vi "输入数据解析.vi"(0 "单个参数补充":dbl, 1 "从板号":dbl=1.0, 2 "主板二维码":string="BNET01", 3 "从板二维码":string="BNET01", 5 "主板引用":refnum<vi>, 7 "从板引用":refnum<vi>, 9 "主板选项":string="三级故障阀值", 11 "枚举":enum16{"主板", "从板"}(ring), 12 "快换":bool caption="快换写入") -> (4 "输出数组":dbl[][](array[numeric]), 6 "数组长度":dbl[](array[numeric]), 8 "循环次数":i32, 10 "命令":u32, 14 "名称":string[](array[string]), 15 "命令序号":u32[](array[numeric]))   [LabVIEW 2013] (continued)
            shift-right: [w13375] -> w13367
            shift-left: dbl[] [] -> [w13371]
            i -> [w13374]
            n5115 = case shown="2" w13374 {
              tunnel: w13373 -> [w13376 w13387 w13398 w13410 w13420 w13431 w13443 w13454]
              tunnel: [w13377 w13388 w13399 w13411 w13422 w13433 w13445 w13455] -> w13372
              frame 0, Default {
                # "最大允许单体电压"
                n5116 = disable-structure shown="启用" {
                  disable-tunnel: [w13383 w13386] -> w13379
                  disable-tunnel: [w13382 w13386] -> w13378
                  disable-tunnel: w13376 -> [w13381 _]
                  frame Disabled {
                    n5117 = Unbundle By Name(w13381) -> ("最大允许单体电压"=w13380:dbl)
                    n5118 = call "输入分辨率计算-EV05.vi"("1字节?"=FALSE, "数值"=w13380, "分辨率"=0.001) -> ("低字节"=w13382:dbl, "高字节1"=w13383:dbl)  [unwired: 2 in, 5 out]
                  }
                  frame Enabled {
                    w13386 = 255 ("高字节1")
                  }
                }
                n5119 = Build Array(w13379, w13378) -> (w13377:i32[])
              }
              frame 1 {
                # "最大允许总电压"
                n5120 = disable-structure shown="启用" {
                  disable-tunnel: [w13394 w13397] -> w13390
                  disable-tunnel: [w13393 w13397] -> w13389
                  disable-tunnel: w13387 -> [w13392 _]
                  frame Disabled {
                    n5121 = Unbundle By Name(w13392) -> ("最大允许总电压"=w13391:dbl)
                    n5122 = call "输入分辨率计算-EV05.vi"("1字节?"=FALSE, "数值"=w13391, "分辨率"=0.1) -> ("低字节"=w13393:dbl, "高字节1"=w13394:dbl)  [unwired: 2 in, 5 out]
                  }
                  frame Enabled {
                    w13397 = 255 ("高字节1")
                  }
                }
                n5123 = Build Array(w13390, w13389) -> (w13388:i32[])
              }
              frame 2 {
                # "最大允许充电电流"
                n5124 = disable-structure shown="启用" {
                  disable-tunnel: [w13406 w13409] -> w13401
                  disable-tunnel: [w13405 w13409] -> w13400
                  disable-tunnel: w13398 -> [w13403 _]
                  frame Enabled {
                    n5125 = Unbundle By Name(w13403) -> ("最大允许充电电流"=w13402:dbl)
                    n5126 = call "输入分辨率计算-EV05.vi"("1字节?"=FALSE, "数值"=w13402, "偏移量"=0.0, "分辨率"=0.1) -> ("低字节"=w13405:dbl, "高字节1"=w13406:dbl)  [unwired: 1 in, 5 out]
                  }
                  frame Disabled {
                    w13409 = 255 ("高字节1")
                  }
                }
                n5127 = Build Array(w13401, w13400) -> (w13399:dbl[])
              }
              frame 3 {
                # "最小允许充电温度"
                n5128 = disable-structure shown="启用" {
                  disable-tunnel: [w13416 255 ("高字节1")] -> w13412
                  disable-tunnel: w13410 -> [w13414 _]
                  frame Disabled {
                    n5129 = Unbundle By Name(w13414) -> ("最小允许温度"=w13413:dbl)
                    n5130 = call "输入分辨率计算-EV05.vi"("1字节?"=TRUE, "数值"=w13413, "偏移量"=-40.0, "分辨率"=1.0) -> ("高字节1"=w13416:dbl)  [unwired: 1 in, 6 out]
                  }
                  frame Enabled {
                  }
                }
                n5131 = Build Array(w13412) -> (w13411:i32[])
              }
              frame 4 {
                # "最小充电电流"
                n5132 = disable-structure shown="启用" {
                  disable-tunnel: [w13427 w13430] -> w13423
                  disable-tunnel: [w13426 w13430] -> w13421
                  disable-tunnel: w13420 -> [w13425 _]
                  frame Disabled {
                    n5133 = Unbundle By Name(w13425) -> ("最小充电电流"=w13424:dbl)
                    n5134 = call "输入分辨率计算-EV05.vi"("1字节?"=FALSE, "数值"=w13424, "分辨率"=0.1) -> ("低字节"=w13426:dbl, "高字节1"=w13427:dbl)  [unwired: 2 in, 5 out]
                  }
                  frame Enabled {
                    w13430 = 255 ("高字节1")
                  }
                }
                n5135 = Build Array(w13423, w13421) -> (w13422:i32[])
              }
              frame 5 {
                # "电流步长"
                n5136 = disable-structure shown="启用" {
                  disable-tunnel: [w13439 w13442] -> w13434
                  disable-tunnel: [w13437 w13442] -> w13432
                  disable-tunnel: w13431 -> [w13436 _]
                  frame Disabled {
                    n5137 = Unbundle By Name(w13436) -> ("电流步长"=w13435:dbl)
                    n5138 = call "输入分辨率计算-EV05.vi"("1字节?"=FALSE, "数值"=w13435, "偏移量"=0.0, "分辨率"=1.0) -> ("低字节"=w13437:dbl, "高字节1"=w13439:dbl)  [unwired: 1 in, 5 out]
                  }
                  frame Enabled {
                    w13442 = 255 ("高字节1")
                  }
                }
                n5139 = Build Array(w13434, w13432) -> (w13433:i32[])
              }
              frame 6 {
                # "最小允许单体电压"
                n5140 = disable-structure shown="启用" {
                  disable-tunnel: [w13450 w13453] -> w13446
                  disable-tunnel: [w13449 w13453] -> w13444
                  disable-tunnel: w13443 -> [w13448 _]
                  frame Disabled {
                    n5141 = Unbundle By Name(w13448) -> ("最小允许单体电压"=w13447:dbl)
                    n5142 = call "输入分辨率计算-EV05.vi"("1字节?"=FALSE, "数值"=w13447, "分辨率"=0.001) -> ("低字节"=w13449:dbl, "高字节1"=w13450:dbl)  [unwired: 2 in, 5 out]
                  }
                  frame Enabled {
                    w13453 = 255 ("高字节1")
                  }
                }
                n5143 = Build Array(w13446, w13444) -> (w13445:i32[])
              }
              frame 7 {
                # "最大允许充电温度"
                n5144 = disable-structure shown="启用" {
                  disable-tunnel: [w13460 255 ("高字节1")] -> w13456
                  disable-tunnel: w13454 -> [w13458 _]
                  frame Disabled {
                    n5145 = Unbundle By Name(w13458) -> ("最大允许充电温度"=w13457:dbl)
                    n5146 = call "输入分辨率计算-EV05.vi"("1字节?"=TRUE, "数值"=w13457, "偏移量"=-40.0, "分辨率"=1.0) -> ("高字节1"=w13460:dbl)  [unwired: 1 in, 6 out]
                  }
                  frame Enabled {
                  }
                }
                n5147 = Build Array(w13456) -> (w13455:i32[])
              }
            }
            n5148 = Insert Into Array(array=w13371, new element=w13372) -> (w13375:dbl[])  [unwired: 1 in]
          }
          n5149 = Build Array(w13367) -> (w13369:dbl[][])
        }
        frame "最小允许充电温度" {
          n5150 = Unbundle By Name(w13467) -> ("充电控制参数"=w13468:refnum<vi>)
          n5151 = property class="Clust (严格)"(reference=w13468) -> ("Value"=w13466:T6)  [unwired: 1 in, 2 out]
          n5152 = for {
            N: 8 -> [_]
            tunnel: w13466 -> [w13478]
            shift-right: [w13480] -> w13472
            shift-left: dbl[] [] -> [w13476]
            i -> [w13479]
            n5153 = case shown="3" w13479 {
              tunnel: w13478 -> [w13481 w13492 w13503 w13515 w13525 w13536 w13548 w13559]
              tunnel: [w13482 w13493 w13504 w13516 w13527 w13538 w13550 w13560] -> w13477
              frame 0, Default {
                # "最大允许单体电压"
                n5154 = disable-structure shown="启用" {
                  disable-tunnel: [w13488 w13491] -> w13484
                  disable-tunnel: [w13487 w13491] -> w13483
                  disable-tunnel: w13481 -> [w13486 _]
                  frame Disabled {
                    n5155 = Unbundle By Name(w13486) -> ("最大允许单体电压"=w13485:dbl)
                    n5156 = call "输入分辨率计算-EV05.vi"("1字节?"=FALSE, "数值"=w13485, "分辨率"=0.001) -> ("低字节"=w13487:dbl, "高字节1"=w13488:dbl)  [unwired: 2 in, 5 out]
                  }
                  frame Enabled {
                    w13491 = 255 ("高字节1")
                  }
                }
                n5157 = Build Array(w13484, w13483) -> (w13482:i32[])
              }
              frame 1 {
                # "最大允许总电压"
                n5158 = disable-structure shown="启用" {
                  disable-tunnel: [w13499 w13502] -> w13495
                  disable-tunnel: [w13498 w13502] -> w13494
                  disable-tunnel: w13492 -> [w13497 _]
                  frame Disabled {
                    n5159 = Unbundle By Name(w13497) -> ("最大允许总电压"=w13496:dbl)
                    n5160 = call "输入分辨率计算-EV05.vi"("1字节?"=FALSE, "数值"=w13496, "分辨率"=0.1) -> ("低字节"=w13498:dbl, "高字节1"=w13499:dbl)  [unwired: 2 in, 5 out]
                  }
                  frame Enabled {
                    w13502 = 255 ("高字节1")
                  }
                }
                n5161 = Build Array(w13495, w13494) -> (w13493:i32[])
              }
              frame 2 {
                # "最大允许充电电流"
                n5162 = disable-structure shown="启用" {
                  disable-tunnel: [w13511 w13514] -> w13506
                  disable-tunnel: [w13510 w13514] -> w13505
                  disable-tunnel: w13503 -> [w13508 _]
                  frame Disabled {
                    n5163 = Unbundle By Name(w13508) -> ("最大允许充电电流"=w13507:dbl)
                    n5164 = call "输入分辨率计算-EV05.vi"("1字节?"=FALSE, "数值"=w13507, "偏移量"=-3000.0, "分辨率"=0.1) -> ("低字节"=w13510:dbl, "高字节1"=w13511:dbl)  [unwired: 1 in, 5 out]
                  }
                  frame Enabled {
                    w13514 = 255 ("高字节1")
                  }
                }
                n5165 = Build Array(w13506, w13505) -> (w13504:i32[])
              }
              frame 3 {
                # "最小允许充电温度"
                n5166 = disable-structure shown="启用" {
                  disable-tunnel: [w13521 255 ("高字节1")] -> w13517
                  disable-tunnel: w13515 -> [w13519 _]
                  frame Enabled {
                    n5167 = Unbundle By Name(w13519) -> ("最小允许充电温度"=w13518:dbl)
                    n5168 = call "输入分辨率计算-EV05.vi"("1字节?"=TRUE, "数值"=w13518, "偏移量"=-40.0, "分辨率"=1.0) -> ("高字节1"=w13521:dbl)  [unwired: 1 in, 6 out]
                  }
                  frame Disabled {
                  }
                }
                n5169 = Build Array(w13517) -> (w13516:dbl[])
              }
              frame 4 {
                # "最小充电电流"
                n5170 = disable-structure shown="启用" {
                  disable-tunnel: [w13532 w13535] -> w13528
                  disable-tunnel: [w13531 w13535] -> w13526
                  disable-tunnel: w13525 -> [w13530 _]
                  frame Disabled {
                    n5171 = Unbundle By Name(w13530) -> ("最小充电电流"=w13529:dbl)
                    n5172 = call "输入分辨率计算-EV05.vi"("1字节?"=FALSE, "数值"=w13529, "分辨率"=0.1) -> ("低字节"=w13531:dbl, "高字节1"=w13532:dbl)  [unwired: 2 in, 5 out]
                  }
                  frame Enabled {
                    w13535 = 255 ("高字节1")
                  }
                }
                n5173 = Build Array(w13528, w13526) -> (w13527:i32[])
              }
              frame 5 {
                # "电流步长"
                n5174 = disable-structure shown="启用" {
                  disable-tunnel: [w13544 w13547] -> w13539
                  disable-tunnel: [w13542 w13547] -> w13537
                  disable-tunnel: w13536 -> [w13541 _]
                  frame Disabled {
                    n5175 = Unbundle By Name(w13541) -> ("电流步长"=w13540:dbl)
                    n5176 = call "输入分辨率计算-EV05.vi"("1字节?"=FALSE, "数值"=w13540, "偏移量"=0.0, "分辨率"=1.0) -> ("低字节"=w13542:dbl, "高字节1"=w13544:dbl)  [unwired: 1 in, 5 out]
                  }
                  frame Enabled {
                    w13547 = 255 ("高字节1")
                  }
                }
                n5177 = Build Array(w13539, w13537) -> (w13538:i32[])
              }
              frame 6 {
                # "最小允许单体电压"
                n5178 = disable-structure shown="启用" {
                  disable-tunnel: [w13555 w13558] -> w13551
                  disable-tunnel: [w13554 w13558] -> w13549
                  disable-tunnel: w13548 -> [w13553 _]
                  frame Disabled {
                    n5179 = Unbundle By Name(w13553) -> ("最小允许单体电压"=w13552:dbl)
                    n5180 = call "输入分辨率计算-EV05.vi"("1字节?"=FALSE, "数值"=w13552, "分辨率"=0.001) -> ("低字节"=w13554:dbl, "高字节1"=w13555:dbl)  [unwired: 2 in, 5 out]
                  }
                  frame Enabled {
                    w13558 = 255 ("高字节1")
                  }
                }
                n5181 = Build Array(w13551, w13549) -> (w13550:i32[])
              }
              frame 7 {
                # "最大允许充电温度"
                n5182 = disable-structure shown="启用" {
                  disable-tunnel: [w13565 255 ("高字节1")] -> w13561
                  disable-tunnel: w13559 -> [w13563 _]
                  frame Disabled {
                    n5183 = Unbundle By Name(w13563) -> ("最大允许充电温度"=w13562:dbl)
                    n5184 = call "输入分辨率计算-EV05.vi"("1字节?"=TRUE, "数值"=w13562, "偏移量"=-40.0, "分辨率"=1.0) -> ("高字节1"=w13565:dbl)  [unwired: 1 in, 6 out]
                  }
                  frame Enabled {
                  }
                }
                n5185 = Build Array(w13561) -> (w13560:i32[])
              }
            }
            n5186 = Insert Into Array(array=w13476, new element=w13477) -> (w13480:dbl[])  [unwired: 1 in]
          }
          n5187 = Build Array(w13472) -> (w13474:dbl[][])
        }
        frame "最小允许充电电流" {
          n5188 = Unbundle By Name(w13572) -> ("充电控制参数"=w13573:refnum<vi>)
          n5189 = property class="Clust (严格)"(reference=w13573) -> ("Value"=w13571:T6)  [unwired: 1 in, 2 out]
          n5190 = for {
            N: 8 -> [_]
            tunnel: w13571 -> [w13583]
            shift-right: [w13585] -> w13577
            shift-left: dbl[] [] -> [w13581]
            i -> [w13584]
            n5191 = case shown="4" w13584 {
              tunnel: w13583 -> [w13586 w13597 w13608 w13620 w13630 w13641 w13653 w13664]
              tunnel: [w13587 w13598 w13609 w13621 w13632 w13643 w13655 w13665] -> w13582
              frame 0, Default {
                # "最大允许单体电压"
                n5192 = disable-structure shown="启用" {
                  disable-tunnel: [w13593 w13596] -> w13589
                  disable-tunnel: [w13592 w13596] -> w13588
                  disable-tunnel: w13586 -> [w13591 _]
                  frame Disabled {
                    n5193 = Unbundle By Name(w13591) -> ("最大允许单体电压"=w13590:dbl)
                    n5194 = call "输入分辨率计算-EV05.vi"("1字节?"=FALSE, "数值"=w13590, "分辨率"=0.001) -> ("低字节"=w13592:dbl, "高字节1"=w13593:dbl)  [unwired: 2 in, 5 out]
                  }
                  frame Enabled {
                    w13596 = 255 ("高字节1")
                  }
                }
                n5195 = Build Array(w13589, w13588) -> (w13587:i32[])
              }
              frame 1 {
                # "最大允许总电压"
                n5196 = disable-structure shown="启用" {
                  disable-tunnel: [w13604 w13607] -> w13600
                  disable-tunnel: [w13603 w13607] -> w13599
                  disable-tunnel: w13597 -> [w13602 _]
                  frame Disabled {
                    n5197 = Unbundle By Name(w13602) -> ("最大允许总电压"=w13601:dbl)
                    n5198 = call "输入分辨率计算-EV05.vi"("1字节?"=FALSE, "数值"=w13601, "分辨率"=0.1) -> ("低字节"=w13603:dbl, "高字节1"=w13604:dbl)  [unwired: 2 in, 5 out]
                  }
                  frame Enabled {
                    w13607 = 255 ("高字节1")
                  }
                }
                n5199 = Build Array(w13600, w13599) -> (w13598:i32[])
              }
              frame 2 {
                # "最大允许充电电流"
                n5200 = disable-structure shown="启用" {
                  disable-tunnel: [w13616 w13619] -> w13611
                  disable-tunnel: [w13615 w13619] -> w13610
                  disable-tunnel: w13608 -> [w13613 _]
                  frame Disabled {
                    n5201 = Unbundle By Name(w13613) -> ("最大允许充电电流"=w13612:dbl)
                    n5202 = call "输入分辨率计算-EV05.vi"("1字节?"=FALSE, "数值"=w13612, "偏移量"=-3000.0, "分辨率"=0.1) -> ("低字节"=w13615:dbl, "高字节1"=w13616:dbl)  [unwired: 1 in, 5 out]
                  }
                  frame Enabled {
                    w13619 = 255 ("高字节1")
                  }
                }
                n5203 = Build Array(w13611, w13610) -> (w13609:i32[])
              }
              frame 3 {
                # "最小允许充电温度"
                n5204 = disable-structure shown="启用" {
                  disable-tunnel: [w13626 255 ("高字节1")] -> w13622
                  disable-tunnel: w13620 -> [w13624 _]
                  frame Disabled {
                    n5205 = Unbundle By Name(w13624) -> ("最小允许温度"=w13623:dbl)
                    n5206 = call "输入分辨率计算-EV05.vi"("1字节?"=TRUE, "数值"=w13623, "偏移量"=-40.0, "分辨率"=1.0) -> ("高字节1"=w13626:dbl)  [unwired: 1 in, 6 out]
                  }
                  frame Enabled {
                  }
                }
                n5207 = Build Array(w13622) -> (w13621:i32[])
              }
              frame 4 {
                # "最小充电电流"
                n5208 = disable-structure shown="启用" {
                  disable-tunnel: [w13637 w13640] -> w13633
                  disable-tunnel: [w13636 w13640] -> w13631
                  disable-tunnel: w13630 -> [w13635 _]
                  frame Enabled {
                    n5209 = Unbundle By Name(w13635) -> ("最小允许充电电流"=w13634:dbl)
                    n5210 = call "输入分辨率计算-EV05.vi"("1字节?"=FALSE, "数值"=w13634, "分辨率"=0.1) -> ("低字节"=w13636:dbl, "高字节1"=w13637:dbl)  [unwired: 2 in, 5 out]
                  }
                  frame Disabled {
                    w13640 = 255 ("高字节1")
                  }
                }
                n5211 = Build Array(w13633, w13631) -> (w13632:dbl[])
              }
              frame 5 {
                # "电流步长"
                n5212 = disable-structure shown="启用" {
                  disable-tunnel: [w13649 w13652] -> w13644
                  disable-tunnel: [w13647 w13652] -> w13642
                  disable-tunnel: w13641 -> [w13646 _]
                  frame Disabled {
                    n5213 = Unbundle By Name(w13646) -> ("电流步长"=w13645:dbl)
                    n5214 = call "输入分辨率计算-EV05.vi"("1字节?"=FALSE, "数值"=w13645, "偏移量"=0.0, "分辨率"=1.0) -> ("低字节"=w13647:dbl, "高字节1"=w13649:dbl)  [unwired: 1 in, 5 out]
                  }
                  frame Enabled {
                    w13652 = 255 ("高字节1")
                  }
                }
                n5215 = Build Array(w13644, w13642) -> (w13643:i32[])
              }
              frame 6 {
                # "最小允许单体电压"
                n5216 = disable-structure shown="启用" {
                  disable-tunnel: [w13660 w13663] -> w13656
                  disable-tunnel: [w13659 w13663] -> w13654
                  disable-tunnel: w13653 -> [w13658 _]
                  frame Disabled {
                    n5217 = Unbundle By Name(w13658) -> ("最小允许单体电压"=w13657:dbl)
                    n5218 = call "输入分辨率计算-EV05.vi"("1字节?"=FALSE, "数值"=w13657, "分辨率"=0.001) -> ("低字节"=w13659:dbl, "高字节1"=w13660:dbl)  [unwired: 2 in, 5 out]
                  }
                  frame Enabled {
                    w13663 = 255 ("高字节1")
                  }
                }
                n5219 = Build Array(w13656, w13654) -> (w13655:i32[])
              }
              frame 7 {
                # "最大允许充电温度"
                n5220 = disable-structure shown="启用" {
                  disable-tunnel: [w13670 255 ("高字节1")] -> w13666
                  disable-tunnel: w13664 -> [w13668 _]
                  frame Disabled {
                    n5221 = Unbundle By Name(w13668) -> ("最大允许充电温度"=w13667:dbl)
                    n5222 = call "输入分辨率计算-EV05.vi"("1字节?"=TRUE, "数值"=w13667, "偏移量"=-40.0, "分辨率"=1.0) -> ("高字节1"=w13670:dbl)  [unwired: 1 in, 6 out]
                  }
                  frame Enabled {
                  }
                }
                n5223 = Build Array(w13666) -> (w13665:i32[])
              }
            }
            n5224 = Insert Into Array(array=w13581, new element=w13582) -> (w13585:dbl[])  [unwired: 1 in]
          }
          n5225 = Build Array(w13577) -> (w13579:dbl[][])
        }
        frame "电流步长" {
          n5226 = Unbundle By Name(w13677) -> ("充电控制参数"=w13678:refnum<vi>)
          n5227 = property class="Clust (严格)"(reference=w13678) -> ("Value"=w13676:T6)  [unwired: 1 in, 2 out]
          n5228 = for {
            N: 8 -> [_]
            tunnel: w13676 -> [w13688]
            shift-right: [w13690] -> w13682
            shift-left: dbl[] [] -> [w13686]
            i -> [w13689]
            n5229 = case shown="5" w13689 {
              tunnel: w13688 -> [w13691 w13702 w13713 w13725 w13735 w13746 w13758 w13769]
              tunnel: [w13692 w13703 w13714 w13726 w13737 w13748 w13760 w13770] -> w13687
              frame 0, Default {
                # "最大允许单体电压"
                n5230 = disable-structure shown="启用" {
                  disable-tunnel: [w13698 w13701] -> w13694
                  disable-tunnel: [w13697 w13701] -> w13693
                  disable-tunnel: w13691 -> [w13696 _]
                  frame Disabled {
                    n5231 = Unbundle By Name(w13696) -> ("最大允许单体电压"=w13695:dbl)
                    n5232 = call "输入分辨率计算-EV05.vi"("1字节?"=FALSE, "数值"=w13695, "分辨率"=0.001) -> ("低字节"=w13697:dbl, "高字节1"=w13698:dbl)  [unwired: 2 in, 5 out]
                  }
                  frame Enabled {
                    w13701 = 255 ("高字节1")
                  }
                }
                n5233 = Build Array(w13694, w13693) -> (w13692:i32[])
              }
              frame 1 {
                # "最大允许总电压"
                n5234 = disable-structure shown="启用" {
                  disable-tunnel: [w13709 w13712] -> w13705
                  disable-tunnel: [w13708 w13712] -> w13704
                  disable-tunnel: w13702 -> [w13707 _]
                  frame Disabled {
                    n5235 = Unbundle By Name(w13707) -> ("最大允许总电压"=w13706:dbl)
                    n5236 = call "输入分辨率计算-EV05.vi"("1字节?"=FALSE, "数值"=w13706, "分辨率"=0.1) -> ("低字节"=w13708:dbl, "高字节1"=w13709:dbl)  [unwired: 2 in, 5 out]
                  }
                  frame Enabled {
                    w13712 = 255 ("高字节1")
                  }
                }
                n5237 = Build Array(w13705, w13704) -> (w13703:i32[])
              }
              frame 2 {
                # "最大允许充电电流"
                n5238 = disable-structure shown="启用" {
                  disable-tunnel: [w13721 w13724] -> w13716
                  disable-tunnel: [w13720 w13724] -> w13715
                  disable-tunnel: w13713 -> [w13718 _]
                  frame Disabled {
                    n5239 = Unbundle By Name(w13718) -> ("最大允许充电电流"=w13717:dbl)
                    n5240 = call "输入分辨率计算-EV05.vi"("1字节?"=FALSE, "数值"=w13717, "偏移量"=-3000.0, "分辨率"=0.1) -> ("低字节"=w13720:dbl, "高字节1"=w13721:dbl)  [unwired: 1 in, 5 out]
                  }
                  frame Enabled {
                    w13724 = 255 ("高字节1")
                  }
                }
                n5241 = Build Array(w13716, w13715) -> (w13714:i32[])
              }
              frame 3 {
                # "最小允许充电温度"
                n5242 = disable-structure shown="启用" {
                  disable-tunnel: [w13731 255 ("高字节1")] -> w13727
                  disable-tunnel: w13725 -> [w13729 _]
                  frame Disabled {
                    n5243 = Unbundle By Name(w13729) -> ("最小允许温度"=w13728:dbl)
                    n5244 = call "输入分辨率计算-EV05.vi"("1字节?"=TRUE, "数值"=w13728, "偏移量"=-40.0, "分辨率"=1.0) -> ("高字节1"=w13731:dbl)  [unwired: 1 in, 6 out]
                  }
                  frame Enabled {
                  }
                }
                n5245 = Build Array(w13727) -> (w13726:i32[])
              }
              frame 4 {
                # "最小充电电流"
                n5246 = disable-structure shown="启用" {
                  disable-tunnel: [w13742 w13745] -> w13738
                  disable-tunnel: [w13741 w13745] -> w13736
                  disable-tunnel: w13735 -> [w13740 _]
                  frame Disabled {
                    n5247 = Unbundle By Name(w13740) -> ("最小充电电流"=w13739:dbl)
                    n5248 = call "输入分辨率计算-EV05.vi"("1字节?"=FALSE, "数值"=w13739, "分辨率"=0.1) -> ("低字节"=w13741:dbl, "高字节1"=w13742:dbl)  [unwired: 2 in, 5 out]
                  }
                  frame Enabled {
                    w13745 = 255 ("高字节1")
                  }
                }
                n5249 = Build Array(w13738, w13736) -> (w13737:i32[])
              }
              frame 5 {
                # "电流步长"
                n5250 = disable-structure shown="启用" {
                  disable-tunnel: [w13754 w13757] -> w13749
                  disable-tunnel: [w13752 w13757] -> w13747
                  disable-tunnel: w13746 -> [w13751 _]
                  frame Enabled {
                    n5251 = Unbundle By Name(w13751) -> ("电流步长"=w13750:dbl)
                    n5252 = call "输入分辨率计算-EV05.vi"("1字节?"=FALSE, "数值"=w13750, "偏移量"=0.0, "分辨率"=0.1) -> ("低字节"=w13752:dbl, "高字节1"=w13754:dbl)  [unwired: 1 in, 5 out]
                  }
                  frame Disabled {
                    w13757 = 255 ("高字节1")
                  }
                }
                n5253 = Build Array(w13749, w13747) -> (w13748:dbl[])
              }
              frame 6 {
                # "最小允许单体电压"
                n5254 = disable-structure shown="启用" {
                  disable-tunnel: [w13765 w13768] -> w13761
                  disable-tunnel: [w13764 w13768] -> w13759
                  disable-tunnel: w13758 -> [w13763 _]
                  frame Disabled {
                    n5255 = Unbundle By Name(w13763) -> ("最小允许单体电压"=w13762:dbl)
                    n5256 = call "输入分辨率计算-EV05.vi"("1字节?"=FALSE, "数值"=w13762, "分辨率"=0.001) -> ("低字节"=w13764:dbl, "高字节1"=w13765:dbl)  [unwired: 2 in, 5 out]
                  }
                  frame Enabled {
                    w13768 = 255 ("高字节1")
                  }
                }
                n5257 = Build Array(w13761, w13759) -> (w13760:i32[])
              }
              frame 7 {
                # "最大允许充电温度"
                n5258 = disable-structure shown="启用" {
                  disable-tunnel: [w13775 255 ("高字节1")] -> w13771
                  disable-tunnel: w13769 -> [w13773 _]
                  frame Disabled {
                    n5259 = Unbundle By Name(w13773) -> ("最大允许充电温度"=w13772:dbl)
                    n5260 = call "输入分辨率计算-EV05.vi"("1字节?"=TRUE, "数值"=w13772, "偏移量"=-40.0, "分辨率"=1.0) -> ("高字节1"=w13775:dbl)  [unwired: 1 in, 6 out]
                  }
                  frame Enabled {
                  }
                }
                n5261 = Build Array(w13771) -> (w13770:i32[])
              }
            }
            n5262 = Insert Into Array(array=w13686, new element=w13687) -> (w13690:dbl[])  [unwired: 1 in]
          }
          n5263 = Build Array(w13682) -> (w13684:dbl[][])
        }
        frame "最小允许单体电压" {
          n5264 = Unbundle By Name(w13782) -> ("充电控制参数"=w13783:refnum<vi>)
          n5265 = property class="Clust (严格)"(reference=w13783) -> ("Value"=w13781:T6)  [unwired: 1 in, 2 out]
          n5266 = for {
            N: 8 -> [_]
            tunnel: w13781 -> [w13793]
            shift-right: [w13795] -> w13787
            shift-left: dbl[] [] -> [w13791]
            i -> [w13794]
            n5267 = case shown="6" w13794 {
              tunnel: w13793 -> [w13796 w13807 w13818 w13830 w13840 w13851 w13863 w13874]
              tunnel: [w13797 w13808 w13819 w13831 w13842 w13853 w13865 w13875] -> w13792
              frame 0, Default {
                # "最大允许单体电压"
                n5268 = disable-structure shown="启用" {
                  disable-tunnel: [w13803 w13806] -> w13799
                  disable-tunnel: [w13802 w13806] -> w13798
                  disable-tunnel: w13796 -> [w13801 _]
                  frame Disabled {
                    n5269 = Unbundle By Name(w13801) -> ("最大允许单体电压"=w13800:dbl)
                    n5270 = call "输入分辨率计算-EV05.vi"("1字节?"=FALSE, "数值"=w13800, "分辨率"=0.001) -> ("低字节"=w13802:dbl, "高字节1"=w13803:dbl)  [unwired: 2 in, 5 out]
                  }
                  frame Enabled {
                    w13806 = 255 ("高字节1")
                  }
                }
                n5271 = Build Array(w13799, w13798) -> (w13797:i32[])
              }
              frame 1 {
                # "最大允许总电压"
                n5272 = disable-structure shown="启用" {
                  disable-tunnel: [w13814 w13817] -> w13810
                  disable-tunnel: [w13813 w13817] -> w13809
                  disable-tunnel: w13807 -> [w13812 _]
                  frame Disabled {
                    n5273 = Unbundle By Name(w13812) -> ("最大允许总电压"=w13811:dbl)
                    n5274 = call "输入分辨率计算-EV05.vi"("1字节?"=FALSE, "数值"=w13811, "分辨率"=0.1) -> ("低字节"=w13813:dbl, "高字节1"=w13814:dbl)  [unwired: 2 in, 5 out]
                  }
                  frame Enabled {
                    w13817 = 255 ("高字节1")
                  }
                }
                n5275 = Build Array(w13810, w13809) -> (w13808:i32[])
              }
              frame 2 {
                # "最大允许充电电流"
                n5276 = disable-structure shown="启用" {
                  disable-tunnel: [w13826 w13829] -> w13821
                  disable-tunnel: [w13825 w13829] -> w13820
                  disable-tunnel: w13818 -> [w13823 _]
                  frame Disabled {
                    n5277 = Unbundle By Name(w13823) -> ("最大允许充电电流"=w13822:dbl)
                    n5278 = call "输入分辨率计算-EV05.vi"("1字节?"=FALSE, "数值"=w13822, "偏移量"=-3000.0, "分辨率"=0.1) -> ("低字节"=w13825:dbl, "高字节1"=w13826:dbl)  [unwired: 1 in, 5 out]
                  }
                  frame Enabled {
                    w13829 = 255 ("高字节1")
                  }
                }
                n5279 = Build Array(w13821, w13820) -> (w13819:i32[])
              }
              frame 3 {
                # "最小允许充电温度"
                n5280 = disable-structure shown="启用" {
                  disable-tunnel: [w13836 255 ("高字节1")] -> w13832
                  disable-tunnel: w13830 -> [w13834 _]
                  frame Disabled {
                    n5281 = Unbundle By Name(w13834) -> ("最小允许温度"=w13833:dbl)
                    n5282 = call "输入分辨率计算-EV05.vi"("1字节?"=TRUE, "数值"=w13833, "偏移量"=-40.0, "分辨率"=1.0) -> ("高字节1"=w13836:dbl)  [unwired: 1 in, 6 out]
                  }
                  frame Enabled {
                  }
                }
                n5283 = Build Array(w13832) -> (w13831:i32[])
              }
              frame 4 {
                # "最小充电电流"
                n5284 = disable-structure shown="启用" {
                  disable-tunnel: [w13847 w13850] -> w13843
                  disable-tunnel: [w13846 w13850] -> w13841
                  disable-tunnel: w13840 -> [w13845 _]
                  frame Disabled {
                    n5285 = Unbundle By Name(w13845) -> ("最小充电电流"=w13844:dbl)
                    n5286 = call "输入分辨率计算-EV05.vi"("1字节?"=FALSE, "数值"=w13844, "分辨率"=0.1) -> ("低字节"=w13846:dbl, "高字节1"=w13847:dbl)  [unwired: 2 in, 5 out]
                  }
                  frame Enabled {
                    w13850 = 255 ("高字节1")
                  }
                }
                n5287 = Build Array(w13843, w13841) -> (w13842:i32[])
              }
              frame 5 {
                # "电流步长"
                n5288 = disable-structure shown="启用" {
                  disable-tunnel: [w13859 w13862] -> w13854
                  disable-tunnel: [w13857 w13862] -> w13852
                  disable-tunnel: w13851 -> [w13856 _]
                  frame Disabled {
                    n5289 = Unbundle By Name(w13856) -> ("电流步长"=w13855:dbl)
                    n5290 = call "输入分辨率计算-EV05.vi"("1字节?"=FALSE, "数值"=w13855, "偏移量"=0.0, "分辨率"=1.0) -> ("低字节"=w13857:dbl, "高字节1"=w13859:dbl)  [unwired: 1 in, 5 out]
                  }
                  frame Enabled {
                    w13862 = 255 ("高字节1")
                  }
                }
                n5291 = Build Array(w13854, w13852) -> (w13853:i32[])
              }
              frame 6 {
                # "最小允许单体电压"
                n5292 = disable-structure shown="启用" {
                  disable-tunnel: [w13870 w13873] -> w13866
                  disable-tunnel: [w13869 w13873] -> w13864
                  disable-tunnel: w13863 -> [w13868 _]
                  frame Enabled {
                    n5293 = Unbundle By Name(w13868) -> ("最小允许单体电压"=w13867:dbl)
                    n5294 = call "输入分辨率计算-EV05.vi"("1字节?"=FALSE, "数值"=w13867, "分辨率"=0.001) -> ("低字节"=w13869:dbl, "高字节1"=w13870:dbl)  [unwired: 2 in, 5 out]
                  }
                  frame Disabled {
                    w13873 = 255 ("高字节1")
                  }
                }
                n5295 = Build Array(w13866, w13864) -> (w13865:dbl[])
              }
              frame 7 {
                # "最大允许充电温度"
                n5296 = disable-structure shown="启用" {
                  disable-tunnel: [w13880 255 ("高字节1")] -> w13876
                  disable-tunnel: w13874 -> [w13878 _]
                  frame Disabled {
                    n5297 = Unbundle By Name(w13878) -> ("最大允许充电温度"=w13877:dbl)
                    n5298 = call "输入分辨率计算-EV05.vi"("1字节?"=TRUE, "数值"=w13877, "偏移量"=-40.0, "分辨率"=1.0) -> ("高字节1"=w13880:dbl)  [unwired: 1 in, 6 out]
                  }
                  frame Enabled {
                  }
                }
                n5299 = Build Array(w13876) -> (w13875:i32[])
              }
            }
            n5300 = Insert Into Array(array=w13791, new element=w13792) -> (w13795:dbl[])  [unwired: 1 in]
          }
          n5301 = Build Array(w13787) -> (w13789:dbl[][])
        }
        frame "最大允许充电温度" {
          n5302 = Unbundle By Name(w13887) -> ("充电控制参数"=w13888:refnum<vi>)
          n5303 = property class="Clust (严格)"(reference=w13888) -> ("Value"=w13886:T6)  [unwired: 1 in, 2 out]
          n5304 = for {
            N: 8 -> [_]
            tunnel: w13886 -> [w13898]
            shift-right: [w13900] -> w13892
            shift-left: dbl[] [] -> [w13896]
            i -> [w13899]
            n5305 = case shown="7" w13899 {
              tunnel: w13898 -> [w13901 w13912 w13923 w13935 w13945 w13956 w13968 w13979]
              tunnel: [w13902 w13913 w13924 w13936 w13947 w13958 w13970 w13980] -> w13897
              frame 0, Default {
                # "最大允许单体电压"
                n5306 = disable-structure shown="启用" {
                  disable-tunnel: [w13908 w13911] -> w13904
                  disable-tunnel: [w13907 w13911] -> w13903
                  disable-tunnel: w13901 -> [w13906 _]
                  frame Disabled {
                    n5307 = Unbundle By Name(w13906) -> ("最大允许单体电压"=w13905:dbl)
                    n5308 = call "输入分辨率计算-EV05.vi"("1字节?"=FALSE, "数值"=w13905, "分辨率"=0.001) -> ("低字节"=w13907:dbl, "高字节1"=w13908:dbl)  [unwired: 2 in, 5 out]
                  }
                  frame Enabled {
                    w13911 = 255 ("高字节1")
                  }
                }
                n5309 = Build Array(w13904, w13903) -> (w13902:i32[])
              }
              frame 1 {
                # "最大允许总电压"
                n5310 = disable-structure shown="启用" {
                  disable-tunnel: [w13919 w13922] -> w13915
                  disable-tunnel: [w13918 w13922] -> w13914
                  disable-tunnel: w13912 -> [w13917 _]
                  frame Disabled {
                    n5311 = Unbundle By Name(w13917) -> ("最大允许总电压"=w13916:dbl)
                    n5312 = call "输入分辨率计算-EV05.vi"("1字节?"=FALSE, "数值"=w13916, "分辨率"=0.1) -> ("低字节"=w13918:dbl, "高字节1"=w13919:dbl)  [unwired: 2 in, 5 out]
                  }
                  frame Enabled {
                    w13922 = 255 ("高字节1")
                  }
                }
                n5313 = Build Array(w13915, w13914) -> (w13913:i32[])
              }
              frame 2 {
                # "最大允许充电电流"
                n5314 = disable-structure shown="启用" {
                  disable-tunnel: [w13931 w13934] -> w13926
                  disable-tunnel: [w13930 w13934] -> w13925
                  disable-tunnel: w13923 -> [w13928 _]
                  frame Disabled {
                    n5315 = Unbundle By Name(w13928) -> ("最大允许充电电流"=w13927:dbl)
                    n5316 = call "输入分辨率计算-EV05.vi"("1字节?"=FALSE, "数值"=w13927, "偏移量"=-3000.0, "分辨率"=0.1) -> ("低字节"=w13930:dbl, "高字节1"=w13931:dbl)  [unwired: 1 in, 5 out]
                  }
                  frame Enabled {
                    w13934 = 255 ("高字节1")
                  }
                }
                n5317 = Build Array(w13926, w13925) -> (w13924:i32[])
              }
              frame 3 {
                # "最小允许充电温度"
                n5318 = disable-structure shown="启用" {
                  disable-tunnel: [w13941 255 ("高字节1")] -> w13937
                  disable-tunnel: w13935 -> [w13939 _]
                  frame Disabled {
                    n5319 = Unbundle By Name(w13939) -> ("最小允许温度"=w13938:dbl)
                    n5320 = call "输入分辨率计算-EV05.vi"("1字节?"=TRUE, "数值"=w13938, "偏移量"=-40.0, "分辨率"=1.0) -> ("高字节1"=w13941:dbl)  [unwired: 1 in, 6 out]
                  }
                  frame Enabled {
                  }
                }
                n5321 = Build Array(w13937) -> (w13936:i32[])
              }
              frame 4 {
                # "最小充电电流"
                n5322 = disable-structure shown="启用" {
                  disable-tunnel: [w13952 w13955] -> w13948
                  disable-tunnel: [w13951 w13955] -> w13946
                  disable-tunnel: w13945 -> [w13950 _]
                  frame Disabled {
                    n5323 = Unbundle By Name(w13950) -> ("最小充电电流"=w13949:dbl)
                    n5324 = call "输入分辨率计算-EV05.vi"("1字节?"=FALSE, "数值"=w13949, "分辨率"=0.1) -> ("低字节"=w13951:dbl, "高字节1"=w13952:dbl)  [unwired: 2 in, 5 out]
                  }
                  frame Enabled {
                    w13955 = 255 ("高字节1")
                  }
                }
                n5325 = Build Array(w13948, w13946) -> (w13947:i32[])
              }
              frame 5 {
                # "电流步长"
                n5326 = disable-structure shown="启用" {
                  disable-tunnel: [w13964 w13967] -> w13959
                  disable-tunnel: [w13962 w13967] -> w13957
                  disable-tunnel: w13956 -> [w13961 _]
                  frame Disabled {
                    n5327 = Unbundle By Name(w13961) -> ("电流步长"=w13960:dbl)
                    n5328 = call "输入分辨率计算-EV05.vi"("1字节?"=FALSE, "数值"=w13960, "偏移量"=0.0, "分辨率"=1.0) -> ("低字节"=w13962:dbl, "高字节1"=w13964:dbl)  [unwired: 1 in, 5 out]
                  }
                  frame Enabled {
                    w13967 = 255 ("高字节1")
                  }
                }
                n5329 = Build Array(w13959, w13957) -> (w13958:i32[])
              }
              frame 6 {
                # "最小允许单体电压"
                n5330 = disable-structure shown="启用" {
                  disable-tunnel: [w13975 w13978] -> w13971
                  disable-tunnel: [w13974 w13978] -> w13969
                  disable-tunnel: w13968 -> [w13973 _]
                  frame Disabled {
                    n5331 = Unbundle By Name(w13973) -> ("最小允许单体电压"=w13972:dbl)
                    n5332 = call "输入分辨率计算-EV05.vi"("1字节?"=FALSE, "数值"=w13972, "分辨率"=0.001) -> ("低字节"=w13974:dbl, "高字节1"=w13975:dbl)  [unwired: 2 in, 5 out]
                  }
                  frame Enabled {
                    w13978 = 255 ("高字节1")
                  }
                }
                n5333 = Build Array(w13971, w13969) -> (w13970:i32[])
              }
              frame 7 {
                # "最大允许充电温度"
                n5334 = disable-structure shown="启用" {
                  disable-tunnel: [w13985 255 ("高字节1")] -> w13981
                  disable-tunnel: w13979 -> [w13983 _]
                  frame Enabled {
                    n5335 = Unbundle By Name(w13983) -> ("最大允许充电温度"=w13982:dbl)
                    n5336 = call "输入分辨率计算-EV05.vi"("1字节?"=TRUE, "数值"=w13982, "偏移量"=-40.0, "分辨率"=1.0) -> ("高字节1"=w13985:dbl)  [unwired: 1 in, 6 out]
                  }
                  frame Disabled {
                  }
                }
                n5337 = Build Array(w13981) -> (w13980:dbl[])
              }
            }
            n5338 = Insert Into Array(array=w13896, new element=w13897) -> (w13900:dbl[])  [unwired: 1 in]
          }
          n5339 = Build Array(w13892) -> (w13894:dbl[][])
        }
        frame "电池信息1" {
          n5340 = Unbundle By Name(w13992) -> ("电池信息"=w13993:refnum<vi>)
          n5341 = property class="Clust (严格)"(reference=w13993) -> ("Value"=w13991:T7)  [unwired: 1 in, 2 out]
          n5342 = for {
            N: 1 -> [_]
            tunnel: [w14002] -> w13997 mode=indexing
            tunnel: [w14001] -> w13996 mode=indexing
            tunnel: [w14003] -> w13994 mode=indexing
            tunnel: w13991 -> [w14000]
            i -> [w13999]
            n5343 = case shown="0, 默认" w13999 {
              tunnel: [30 ("单个参数补充") 4 ("单个参数补充") 8 ("单个参数补充") 6 ("单个参数补充")] -> w14002
              tunnel: [1 ("命令序号") 2 ("命令序号") 3 ("命令序号") 4 ("命令序号")] -> w14001
              tunnel: [w14052 w14098 w14124 w14136] -> w14003
              tunnel: w14000 -> [w14053 w14097 w14107 w14130]
              frame 0, Default {
                w14060 = 2 ("偏移量(0)")
                w14013 = ":" ("正则表达式")
                w14021 = 0.0 ("元素")
                w14040 = 256.0 ("y")
                w14045 = 256.0 ("y")
                w14057 = "-" ("正则表达式")
                n5344 = Unbundle By Name(w14053) -> ("电池包额定能量"=w14026:dbl, "电池包额定容量"=w14028:dbl, "实际容量"=w14027:dbl, "电池包额定总电压"=w14051:dbl)
                n5345 = Unbundle By Name(w14053) -> ("电池串联"=w14068:dbl, "电池并联"=w14067:dbl, "电池厂家"=w14066:string, "电池类型"=w14064:string, "电池生产日期"=w14062:string)
                n5346 = Match Pattern(string=w14062, regular expression=w14057) -> (before substring=w14061:string, after substring=w14058:string)  [unwired: 3 out]
                n5347 = Match Pattern(string=w14058, regular expression=w14057) -> (before substring=w14056:string, after substring=w14019:string)  [unwired: 3 out]
                n5348 = Match Pattern(string=w14019, regular expression=" " ("正则表达式")) -> (before substring=w14017:string, after substring=w14016:string)  [unwired: 3 out]
                n5349 = call "输入分辨率计算-EV05.vi"("1字节?"=FALSE, "数值"=w14026, "分辨率"=0.1) -> ("低字节"=w14025:dbl, "高字节1"=w14024:dbl)  [unwired: 2 in, 5 out]
                n5350 = String Subset(string=w14061, offset (0)=w14060, length (rest)=w14060) -> (substring=w14059:string)
                n5351 = call "输入分辨率计算-EV05.vi"("1字节?"=TRUE, "数值 2"=w14027, "数值"=w14028, "分辨率"=0.001) -> ("高字节 2"=w14029:dbl, "高字节1"=w14030:dbl)  [unwired: 1 in, 5 out]
                n5352 = Match Pattern(string=w14016, regular expression=w14013) -> (before substring=w14015:string, after substring=w14014:string)  [unwired: 3 out]
                n5353 = Fract/Exp String To Number(string=w14059) -> (number=w14009:dbl)  [unwired: 1 in, 3 out]
                n5354 = Fract/Exp String To Number(string=w14056) -> (number=w14008:dbl)  [unwired: 4 out]
                n5355 = Fract/Exp String To Number(string=w14017) -> (number=w14007:dbl)  [unwired: 4 out]
                n5356 = case shown="\"2\", \"盟固利\"" w14066 {
                  tunnel: [2 1] -> w14065
                  frame "2", "盟固利" {
                  }
                  frame "1", "普莱德", Default {
                  }
                }
                n5357 = case shown="\"9\", \"其他电池\"" w14064 {
                  tunnel: [2 3 4 5 6 7 8 9 1] -> w14063
                  frame "2", "锰酸锂" {
                  }
                  frame "3", "三元材料" {
                  }
                  frame "4", "铅酸" {
                  }
                  frame "5", "镍氢" {
                  }
                  frame "6", "钴酸锂" {
                  }
                  frame "7", "聚合物锂离子" {
                  }
                  frame "8", "钛酸锂" {
                  }
                  frame "9", "其他电池" {
                  }
                  frame "1", "磷酸铁锂", Default {
                  }
                }
                n5358 = Match Pattern(string=w14014, regular expression=w14013) -> (before substring=w14012:string, after substring=w14011:string)  [unwired: 3 out]
                n5359 = call "输入分辨率计算-EV05.vi"("1字节?"=FALSE, "数值"=w14051, "分辨率"=0.1) -> ("低字节"=w14022:dbl, "高字节1"=w14023:dbl)  [unwired: 2 in, 5 out]
                n5360 = Quotient & Remainder(x=w14030, y=w14045) -> (x-y*floor(x/y)=w14044:dbl, floor(x/y)=w14048:dbl)
                n5361 = Fract/Exp String To Number(string=w14015) -> (number=w14006:dbl)  [unwired: 4 out]
                n5362 = Quotient & Remainder(x=w14029, y=w14040) -> (x-y*floor(x/y)=w14036:dbl, floor(x/y)=w14037:dbl)
                n5363 = Quotient & Remainder(x=w14048, y=w14045) -> (x-y*floor(x/y)=w14043:dbl, floor(x/y)=w14047:dbl)
                n5364 = Fract/Exp String To Number(string=w14012) -> (number=w14005:dbl)  [unwired: 4 out]
                n5365 = Quotient & Remainder(x=w14037, y=w14040) -> (x-y*floor(x/y)=w14035:dbl, floor(x/y)=w14038:dbl)
                n5366 = call <vilib>:"Trim Whitespace.vi"("string"=w14011) -> ("trimmed string"=w14010:string)  [unwired: 1 in]
                n5367 = Quotient & Remainder(x=w14047, y=w14045) -> (x-y*floor(x/y)=w14042:dbl, floor(x/y)=w14046:dbl)
                n5368 = Quotient & Remainder(x=w14038, y=w14040) -> (x-y*floor(x/y)=w14034:dbl, floor(x/y)=w14039:dbl)
                n5369 = Quotient & Remainder(x=w14068, y=256.0) -> (x-y*floor(x/y)=w14070:dbl, floor(x/y)=w14071:dbl)
                n5370 = Fract/Exp String To Number(string=w14010) -> (number=w14004:dbl)  [unwired: 4 out]
                n5371 = Quotient & Remainder(x=w14046, y=w14045) -> (x-y*floor(x/y)=w14041:dbl)  [unwired: 1 out]
                n5372 = Quotient & Remainder(x=w14039, y=w14040) -> (x-y*floor(x/y)=w14033:dbl)  [unwired: 1 out]
                n5373 = Build Array(w14024, w14025, w14041, w14042, w14043, w14044, w14033, w14034, w14035, w14036, w14023, w14022, w14021, w14021, w14021, w14009, w14008, w14007, w14006, w14005, w14004) -> (w14020:dbl[])
                n5374 = Build Array(w14071, w14070, w14067, w14065, w14063) -> (w14069:dbl[])
                n5375 = Insert Into Array(array=w14069, new element=w14020) -> (w14052:dbl[])  [unwired: 1 in]
              }
              frame 1 {
                w14088 = 256.0 ("y")
                n5376 = Unbundle By Name(w14097) -> ("电池包组号"=w14096:string)
                n5377 = Match Pattern(string=w14096, regular expression="-" ("正则表达式")) -> (before substring=w14094:string, after substring=w14093:string)  [unwired: 3 out]
                n5378 = Fract/Exp String To Number(string=w14094) -> (number=w14092:dbl)  [unwired: 1 in, 3 out]
                n5379 = Fract/Exp String To Number(string=w14093) -> (number=w14089:dbl)  [unwired: 4 out]
                n5380 = Quotient & Remainder(x=w14089, y=w14088) -> (x-y*floor(x/y)=w14086:dbl, floor(x/y)=w14087:dbl)
                n5381 = Quotient & Remainder(x=w14092, y=w14088) -> (x-y*floor(x/y)=w14090:dbl, floor(x/y)=w14091:dbl)
                n5382 = Build Array(w14091, w14090, w14087, w14086) -> (w14098:dbl[])
              }
              frame 2 {
                w14115 = 256.0 ("y")
                w14120 = 256.0 ("y")
                n5383 = Unbundle By Name(w14107) -> ("累计充电总安时"=w14104:dbl, "累计放电总安时"=w14103:dbl)
                n5384 = call "输入分辨率计算-EV05.vi"("1字节?"=TRUE, "数值 2"=w14103, "数值"=w14104, "分辨率"=0.001) -> ("高字节 2"=w14101:dbl, "高字节1"=w14102:dbl)  [unwired: 1 in, 5 out]
                n5385 = Quotient & Remainder(x=w14102, y=w14120) -> (x-y*floor(x/y)=w14119:dbl, floor(x/y)=w14123:dbl)
                n5386 = Quotient & Remainder(x=w14101, y=w14115) -> (x-y*floor(x/y)=w14111:dbl, floor(x/y)=w14112:dbl)
                n5387 = Quotient & Remainder(x=w14123, y=w14120) -> (x-y*floor(x/y)=w14118:dbl, floor(x/y)=w14122:dbl)
                n5388 = Quotient & Remainder(x=w14112, y=w14115) -> (x-y*floor(x/y)=w14110:dbl, floor(x/y)=w14113:dbl)
                n5389 = Quotient & Remainder(x=w14122, y=w14120) -> (x-y*floor(x/y)=w14117:dbl, floor(x/y)=w14121:dbl)
                n5390 = Quotient & Remainder(x=w14113, y=w14115) -> (x-y*floor(x/y)=w14109:dbl, floor(x/y)=w14114:dbl)
                n5391 = Quotient & Remainder(x=w14121, y=w14120) -> (x-y*floor(x/y)=w14116:dbl)  [unwired: 1 out]
                n5392 = Quotient & Remainder(x=w14114, y=w14115) -> (x-y*floor(x/y)=w14108:dbl)  [unwired: 1 out]
                n5393 = Build Array(w14116, w14117, w14118, w14119, w14108, w14109, w14110, w14111) -> (w14124:dbl[])
              }
              frame 3 {
                w14135 = 256.0 ("y")
                n5394 = Unbundle By Name(w14130) -> ("电池放空次数"=w14129:dbl, "电池充满次数"=w14128:dbl, "电池充电次数"=w14127:dbl)
                n5395 = Quotient & Remainder(x=w14129, y=w14135) -> (x-y*floor(x/y)=w14137:dbl, floor(x/y)=w14138:dbl)
                n5396 = Quotient & Remainder(x=w14128, y=w14135) -> (x-y*floor(x/y)=w14133:dbl, floor(x/y)=w14134:dbl)
                n5397 = Quotient & Remainder(x=w14127, y=w14135) -> (x-y*floor(x/y)=w14131:dbl, floor(x/y)=w14132:dbl)
                n5398 = Build Array(w14138, w14137, w14134, w14133, w14132, w14131) -> (w14136:dbl[])
              }
            }
          }
        }
        frame "电池信息" {
          n5399 = Unbundle By Name(w14144) -> ("电池信息"=w14145:refnum<vi>)
          n5400 = property class="Clust (严格)"(reference=w14145) -> ("Value"=w14143:T7)  [unwired: 1 in, 2 out]
          n5401 = for {
            N: 4 -> [_]
            tunnel: [w14156] -> w14149 mode=indexing
            tunnel: [w14155] -> w14148 mode=indexing
            tunnel: [w14153] -> w14146 mode=indexing
            tunnel: w14143 -> [w14152]
            tunnel: [w14151] -> w14141 mode=indexing
            i -> [w14154]
            n5402 = case shown="1" w14154 {
              tunnel: [30 ("单个参数补充") 4 ("单个参数补充") 8 ("单个参数补充") 6 ("单个参数补充")] -> w14156
              tunnel: [1 ("命令序号") 2 ("命令序号") 3 ("命令序号") 4 ("命令序号")] -> w14155
              tunnel: [w14206 w14240 w14280 w14293] -> w14153
              tunnel: w14152 -> [w14207 w14241 w14263 w14287]
              tunnel: ["电池组信息1" "电池包组号" "充放电安时" "电池充放电次数"] -> w14151
              frame 0, Default {
                w14214 = 2 ("偏移量(0)")
                w14166 = ":" ("正则表达式")
                w14174 = 0.0 ("元素")
                w14193 = 256.0 ("y")
                w14198 = 256.0 ("y")
                w14211 = "-" ("正则表达式")
                n5403 = Unbundle By Name(w14207) -> ("电池包额定能量"=w14179:dbl, "电池包额定容量"=w14181:dbl, "实际容量"=w14180:dbl, "电池包额定总电压"=w14204:dbl)
                n5404 = Unbundle By Name(w14207) -> ("电池串联"=w14222:dbl, "电池并联"=w14221:dbl, "电池厂家"=w14220:string, "电池类型"=w14218:string, "电池生产日期"=w14216:string)
                n5405 = Match Pattern(string=w14216, regular expression=w14211) -> (before substring=w14215:string, after substring=w14212:string)  [unwired: 3 out]
                n5406 = Match Pattern(string=w14212, regular expression=w14211) -> (before substring=w14210:string, after substring=w14172:string)  [unwired: 3 out]
                n5407 = Match Pattern(string=w14172, regular expression=" " ("正则表达式")) -> (before substring=w14170:string, after substring=w14169:string)  [unwired: 3 out]
                n5408 = call "输入分辨率计算-EV05.vi"("1字节?"=FALSE, "数值"=w14179, "分辨率"=0.1) -> ("低字节"=w14178:dbl, "高字节1"=w14177:dbl)  [unwired: 2 in, 5 out]
                n5409 = String Subset(string=w14215, offset (0)=w14214, length (rest)=w14214) -> (substring=w14213:string)
                n5410 = call "输入分辨率计算-EV05.vi"("1字节?"=TRUE, "数值 2"=w14180, "数值"=w14181, "分辨率"=0.001) -> ("高字节 2"=w14182:dbl, "高字节1"=w14183:dbl)  [unwired: 1 in, 5 out]
                n5411 = Match Pattern(string=w14169, regular expression=w14166) -> (before substring=w14168:string, after substring=w14167:string)  [unwired: 3 out]
                n5412 = Fract/Exp String To Number(string=w14213) -> (number=w14162:dbl)  [unwired: 1 in, 3 out]
                n5413 = Fract/Exp String To Number(string=w14210) -> (number=w14161:dbl)  [unwired: 4 out]
                n5414 = Fract/Exp String To Number(string=w14170) -> (number=w14160:dbl)  [unwired: 4 out]
                n5415 = case shown="\"2\", \"盟固利\"" w14220 {
                  tunnel: [2 1] -> w14219
                  frame "2", "盟固利" {
                  }
                  frame "1", "普莱德", Default {
                  }
                }
                n5416 = case shown="\"9\", \"其他电池\"" w14218 {
                  tunnel: [2 3 4 5 6 7 8 9 1] -> w14217
                  frame "2", "锰酸锂" {
                  }
                  frame "3", "三元材料" {
                  }
